vi "GetExplanation.vi"(9 "Error in":errorcluster) -> (1 "Explanation":string)   [LabVIEW 2017, in "GPError.lvlib"]
doc: "Returns <B>Explanation</B> derived from <B>Error in</B>, just like when you right click on an error cluster indicator and select 'Explain Error' or 'Explain Warning'. For appended errors the explanation from the primary error/warning is returned only.\n\nThis VI is inlined.\n\nSteen Schmidt\nGPower\n17/7 2013"
uses:
  GPError.lvlib
  <vilib>/Utility/error.llb/DialogType.ctl
panel:
  # "Copyright © 2013\nSteen Schmidt, GPower\nSee enclosed license file for terms and conditions"
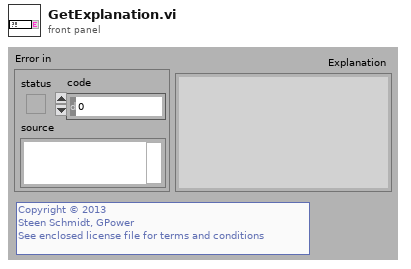
[diagram p1: front panel]
types:
  T1 = typedef "DialogType.ctl" = u16
  T2 = typedef "GPError.lvlib/ErrorType.ctl" = enum16{"No Error", "Error", "Warning", "Appended errors", "Appended warnings", "Appended mixed"}
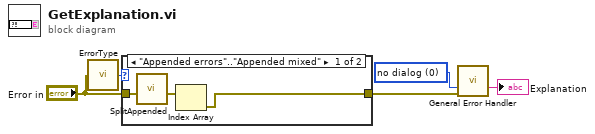
[diagram p0: block diagram]
diagram:
  w5 = T1 0 items=["no dialog", "OK message", "continue or stop message", "OK message + warnings", "continue/stop + warnings"] ("type of dialog (OK msg:1)")
  n1 = call "ErrorType.vi"("Error in"="Error in") -> ("Error type"=w3:T2)  [unwired: 4 in]
  n2 = case shown="\"Appended errors\"..\"Appended mixed\"" w3 {
    tunnel: "Error in" -> [w8 w9]
    tunnel: [w6 w9] -> w1
    frame "Appended errors".."Appended mixed" {
      n3 = call "SplitAppended.vi"("Appended errors in"=w8) -> ("Errors out"=w7:errorcluster[])  [unwired: 10 in]
      n4 = Index Array(array=w7) -> (element=w6:errorcluster)  [unwired: 1 in]
    }
    frame "No Error".."Warning" {
    }
  }
  n5 = call <vilib>:"General Error Handler.vi"("type of dialog (OK msg:1)"=w5, "error in (no error)"=w1) -> ("message"=→"Explanation":string)  [unwired: 9 in, 4 out]
